vi "Save-Recall Setup.vi"(7 "Setup(0:Instrument Setup)":u16(ring) items=["Instrument Setup", "List Setup"], 8 "error in (no error)":errorcluster, 9 "Memory Address(1)":dbl=1.0, 10 "Action(0:Save)":u16(ring) items=["Save", "Recall"], 11 "VISA resource name":refnum<visa-resource-name>) -> (0 "error out":errorcluster, 3 "VISA resource name out":refnum<visa-resource-name>)   [LabVIEW 2021, in "Keithley 2200 Series.lvlib"]
doc: "Save or recall instrument settings to or from memory (parameter: 1~7).\nExample: LIST:SAV 1 or LIST:RCL 1"
uses:
  <instrlib>/Keithley 2200 Series/Keithley 2200 Series.lvlib
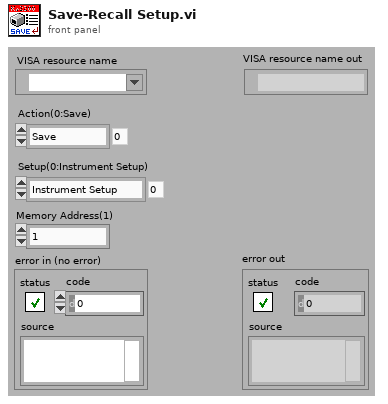
[diagram p1: front panel]
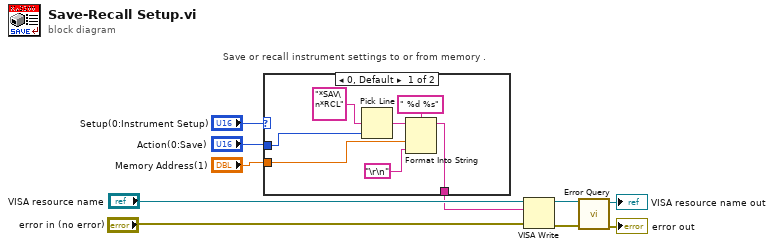
[diagram p0: block diagram]
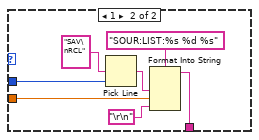
[diagram p2: hidden frame]
diagram:
  # "Save or recall instrument settings to or from memory ."
  n1 = case shown="0, Default" "Setup(0:Instrument Setup)" {
    tunnel: [w13 w22] -> w4
    tunnel: "Action(0:Save)" -> [w12 w19]
    tunnel: "Memory Address(1)" -> [w11 w18]
    frame 0, Default {
      n2 = Pick Line(multi-line string="*SAV\n*RCL", line index=w12) -> (output string=w16:string)  [unwired: 1 out]
      n3 = Format Into String(format string=" %d %s", initial string=w16, w11, "\r\n") -> (resulting string=w13:string)  [unwired: 1 in, 1 out]
    }
    frame 1 {
      n4 = Pick Line(multi-line string="SAV\nRCL", line index=w19) -> (output string=w21:string)  [unwired: 1 out]
      n5 = Format Into String(format string="SOUR:LIST:%s %d %s", w21, w18, "\r\n") -> (resulting string=w22:string)  [unwired: 2 in, 1 out]
    }
  }
  n6 = VISA Write(VISA resource name="VISA resource name", write buffer=w4, error in (no error)="error in (no error)") -> (VISA resource name out=w8:refnum<visa-resource-name>, error out=w7:errorcluster)  [unwired: 1 out]
  n7 = call <instrlib>:"Error Query.vi"("error in (no error)"=w7, "VISA resource name"=w8) -> ("error out"=→"error out":errorcluster, "VISA resource name out"=→"VISA resource name out":refnum<visa-resource-name>)  [unwired: 8 out]
